vi "GetControlImage.vi"(0 "Control ref":refnum<vi>, 5 "error in (no error)":errorcluster) -> (14 "base64 encoded <img> string 1":string, 16 "base64 encoded <img> string 2":string, 19 "error out":errorcluster)   [LabVIEW 2014, in "FrontPanelPublisher.lvlib" / "Control.lvclass"]
uses:
  Control.lvclass
  FrontPanelPublisher.lvlib
  <vilib>/wsapi/NI_WebServices.lvlib
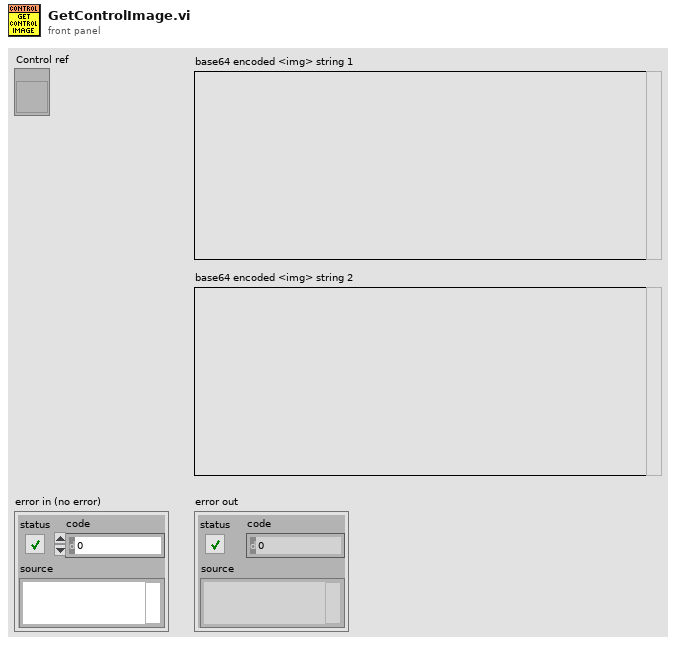
[diagram p1: front panel]
types:
  T1 = typedef "imagedata.ctl" = cluster{"image type":i32, "image depth":i32, "image":u8[], "mask":u8[], "colors":u32[], "Rectangle":cluster{"left":i16, "top":i16, "right":i16, "bottom":i16}}
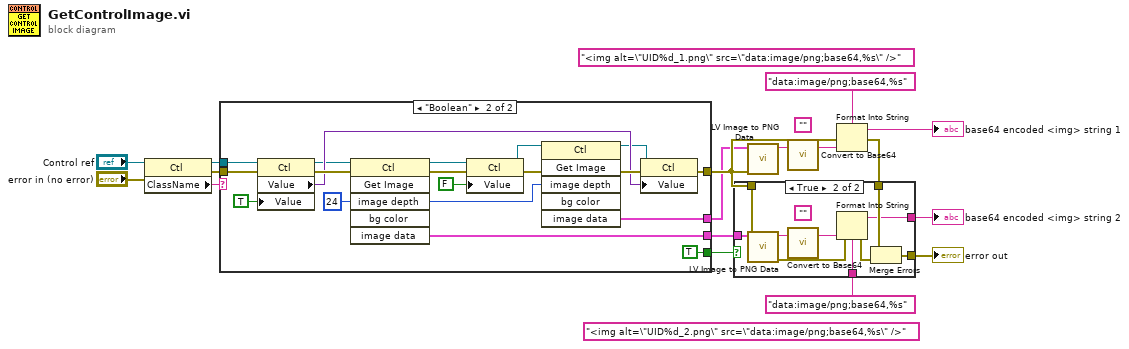
[diagram p0: block diagram]
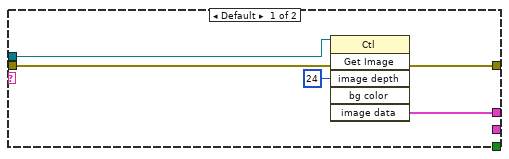
[diagram p3: hidden frame]
diagram:
  (unwired) "<img alt=\"UID%d_2.png\" src=\"data:image/png;base64,%s\" />" ("string")
  (unwired) "<img alt=\"UID%d_1.png\" src=\"data:image/png;base64,%s\" />" ("string")
  (unwired) ""
  n1 = property on="Property Node" class="Ctl"(reference="Control ref", error in="error in (no error)") -> (reference out=w11:refnum<vi>, error out=w16:errorcluster, "ClassName"=w10:string)
  n2 = case shown="\"Boolean\"" w10 {
    tunnel: [_ w24] -> w4
    tunnel: [w18 w25] -> w7
    tunnel: [w21 w36] -> w13
    tunnel: w11 -> [w19 w26]
    tunnel: w16 -> [w22 w35]
    tunnel: [_ TRUE ("Value")] -> w1
    frame Default {
      n3 = invoke on="Invoke Node" class="Ctl" method="Get Image"(reference=w19, error in=w22, "image depth"=24 ("Image Depth")) -> (error out=w21:errorcluster, "image data"=w18:T1)  [unwired: 3 in, 4 out]
    }
    frame "Boolean" {
      w27 = 24 ("Image Depth")
      n4 = property on="Property Node" class="Ctl"(reference=w26, error in=w35, "Value"=TRUE) -> (reference out=w31:refnum<vi>, error out=w37:errorcluster, "Value"=w34:variant)
      n5 = invoke on="Invoke Node" class="Ctl" method="Get Image"(reference=w31, error in=w37, "image depth"=w27) -> (reference out=w30:refnum<vi>, error out=w38:errorcluster, "image data"=w24:T1)  [unwired: 3 in, 3 out]
      n6 = property on="Property Node" class="Ctl"(reference=w30, error in=w38, "Value"=FALSE) -> (reference out=w33:refnum<vi>, error out=w40:errorcluster)
      n7 = invoke on="Invoke Node" class="Ctl" method="Get Image"(reference=w33, error in=w40, "image depth"=w27) -> (reference out=w32:refnum<vi>, error out=w39:errorcluster, "image data"=w25:T1)  [unwired: 3 in, 3 out]
      n8 = property on="Property Node" class="Ctl"(reference=w32, error in=w39, "Value"=w34) -> (error out=w36:errorcluster)  [unwired: 1 out]
    }
  }
  n9 = call <vilib>:"LV Image to PNG Data.vi"("error in (no error)"=w13, "image data"=w7) -> ("png data"=w6:string)  [unwired: 8 in, 1 out]
  n10 = call "Convert to Base64.vi"("String"=w6) -> ("Base64 String"=w9:string)  [unwired: 2 in]
  n11 = Format Into String(format string="data:image/png;base64,%s" ("string"), error in=w13, w9) -> (resulting string=→"base64 encoded <img> string 1":string, error out=w15:errorcluster)  [unwired: 1 in]
  n12 = case shown="True" w1 {
    tunnel: w15 -> [w41 w51]
    tunnel: [w41 w49] -> w14
    tunnel: w13 -> [_ w47]
    tunnel: "data:image/png;base64,%s" ("string") -> [_ w45]
    tunnel: w4 -> [_ w43]
    tunnel: [_ w42] -> w2
    frame False {
    }
    frame True {
      (unwired) ""
      n13 = call <vilib>:"LV Image to PNG Data.vi"("error in (no error)"=w47, "image data"=w43) -> ("error out"=w50:errorcluster, "png data"=w46:string)  [unwired: 8 in]
      n14 = call "Convert to Base64.vi"("String"=w46) -> ("Base64 String"=w44:string)  [unwired: 2 in]
      n15 = Format Into String(format string=w45, error in=w50, w44) -> (resulting string=w42:string, error out=w48:errorcluster)  [unwired: 1 in]
      n16 = Merge Errors(w51, w48) -> (w49:errorcluster)
    }
  }
  "error out" <- w14
  "base64 encoded <img> string 2" <- w2
